vi "DAQ.GenerateWaveform.vi"(8 "error in (no error)":errorcluster, 11 "DAQ in":refnum<class "DAQ.lvclass">) -> (0 "error out":errorcluster, 2 "Waveforms":waveform(dbl)[](array[waveform]), 3 "DAQ out":refnum<class "DAQ.lvclass">)   [LabVIEW 2016, in "DAQ.lvclass"]
uses:
  DAQ.lvclass
  DAQ.lvclass/DAQ.ctl
  <vilib>/measure/NI_MABase.lvlib
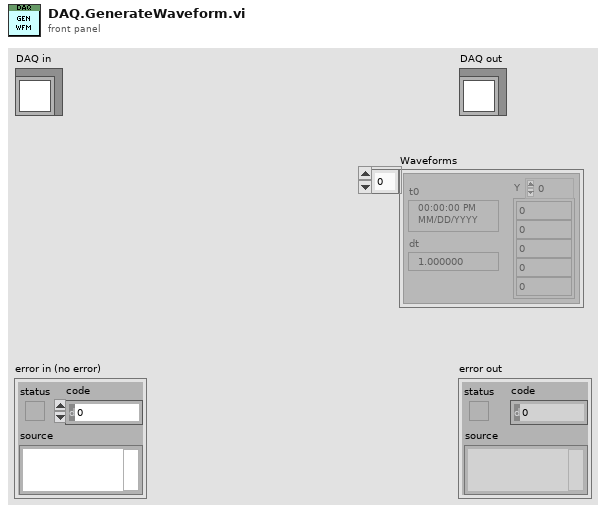
[diagram p1: front panel]
types:
  T1 = typedef "DAQ.lvclass/PrivateEvents--DAQ.AI.Channels.ctl" = string
  T2 = typedef "DAQ.lvclass/DAQ_SamplingInfo.ctl" = cluster{"Fs":dbl, "#s":dbl}
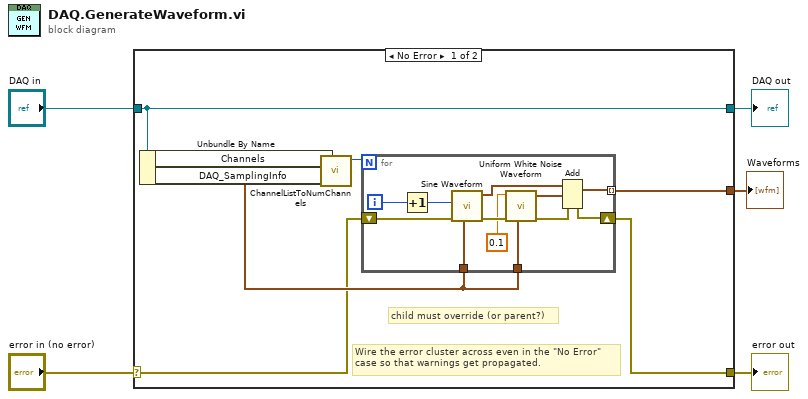
[diagram p0: block diagram]
diagram:
  n1 = case shown="No Error" "error in (no error)" {
    selector: "error in (no error)" -> [w6 w26]
    tunnel: [w7 w26] -> w1
    tunnel: [w11 w25] -> w3
    tunnel: "DAQ in" -> [w11 w25]
    tunnel: [w12 _] -> w2
    frame No Error {
      # "child must override (or parent?)"
      # "Wire the error cluster across even in the \"No Error\"\ncase so that warnings get propagated."
      n2 = Unbundle By Name(w11) -> ("Channels"=w9:T1, "DAQ_SamplingInfo"=w8:T2)
      n3 = call "ChannelListToNumChannels.vi"("Channels"=w9) -> ("Numeric"=w10:i32)  [unwired: 10 in]
      n4 = for {
        N: w10 -> [_]
        tunnel: [w20] -> w12 mode=indexing
        tunnel: w8 -> [w18]
        tunnel: w8 -> [w17]
        shift-right: [w14] -> w7
        shift-left: w6 -> [w13]
        i -> [w24]
        n5 = Increment(x=w24) -> (x+1=w16:i32)
        n6 = call <vilib>:"Sine Waveform.vi"("sampling info"=w18, "error in (no error)"=w13, "amplitude"=w16) -> ("error out"=w23:errorcluster, "signal out"=w21:waveform(dbl))  [unwired: 7 in]
        n7 = call <vilib>:"Uniform White Noise Waveform.vi"("sampling info"=w17, "error in (no error)"=w23, "amplitude"=0.1) -> ("error out"=w15:errorcluster, "signal out"=w22:waveform(dbl))  [unwired: 7 in]
        n8 = Add(1:w22, 2:w21, 4:w15) -> (0:w20:waveform(dbl), 3:w14:errorcluster)
      }
    }
    frame Error {
    }
  }
  "error out" <- w1
  "DAQ out" <- w3
  "Waveforms" <- w2
